vi "Prep_Config_Files_Tomography_v1.vi"() -> ()   [LabVIEW 2021]
uses:
  Pulses_char.ctl
  Drivers/Arduino_Pulse_Generator/Configurate/Channel_Pulse_Stream.ctl
  Drivers/Arduino_Pulse_Generator/Configurate/Register_1.ctl
  Drivers/Arduino_Pulse_Generator/Configurate/Register_2.ctl
  b441c710-b50f-4b81-872d-f4532ec974e2.vi
  <vilib>/Comparison/Less/Less Functor/Less Functor.lvclass
panel:
  in  "Additional mag field pumping pulse 4":T1={"Times"=[140010.0, 140020.0], "channel"=12} {"channel" min=2 max=13 step=1}
  in  "Additional mag field pumping pulse 3":T1={"Times"=[140010.0, 140020.0], "channel"=12} {"channel" min=2 max=13 step=1}
  in  "Additional mag field pumping pulse 2":T1={"Times"=[140010.0, 140020.0], "channel"=12} {"channel" min=2 max=13 step=1}
  in  "Additional mag field pumping pulse":T1={"Times"=[140010.0, 140020.0], "channel"=12} {"channel" min=2 max=13 step=1}
  out "Array - Numeric":dbl[][][][](array[numeric])
  out "Keithley TRIG":T1={"Times"=[], "channel"=2} {"channel" min=2 max=13 step=1}
  out "post_control_zy":T1={"Times"=[], "channel"=2} {"channel" min=2 max=13 step=1}
  out "post_control_non":T1={"Times"=[], "channel"=2} {"channel" min=2 max=13 step=1}
  out "post_control_y":T1={"Times"=[], "channel"=2} {"channel" min=2 max=13 step=1}
  out "post_control_z":T1={"Times"=[], "channel"=2} {"channel" min=2 max=13 step=1}
  out "control_3":T1={"Times"=[], "channel"=2} {"channel" min=2 max=13 step=1}
  out "control_2":T1={"Times"=[], "channel"=2} {"channel" min=2 max=13 step=1}
  out "control_1":T1={"Times"=[], "channel"=2} {"channel" min=2 max=13 step=1}
  out "post_cont_pulse_length":dbl
  out "control_pulse_length":dbl
  out "probe_start":dbl
  out "pump_end":dbl
  in  "Probing optical beam \nchannel":u8=2 min=2 max=13 step=1
  in  "Accqusition TRIG \nchannel":u8=6 min=2 max=13 step=1
  in  "Pumping magnetic field":T1={"Times"=[39995.0, 140005.0], "channel"=8} {"channel" min=2 max=13 step=1}
  in  "Z coil\nchannel":u8=10 min=2 max=13 step=1
  in  "Y coil\nchannel":u8=9 min=2 max=13 step=1
  in  "X coil \nchannel":u8=8 min=2 max=13 step=1
  in  "Keithley preTRIG":T1={"Times"=[2000.0, 3000.0], "channel"=5} {"channel" min=2 max=13 step=1}
  out "Accquisition TRIG":T1={"Times"=[], "channel"=2} {"channel" min=2 max=13 step=1}
  in  "Keithley ARM":T1={"Times"=[0.0, 1000.0], "channel"=4} {"channel" min=2 max=13 step=1}
  out "Probing optical beam":T1={"Times"=[], "channel"=2} {"channel" min=2 max=13 step=1}
  in  "Repumping optical beam":T1={"Times"=[40000.0, 140000.0], "channel"=3} {"channel" min=2 max=13 step=1}
  in  "Pumping optical beam":T1={"Times"=[40000.0, 140000.0], "channel"=7} {"channel" min=2 max=13 step=1}
  out "Pulses_char [ms]":T2
  in  "Z pi pulse [us]":dbl=68.0
  in  "Y pi pulse [us]":dbl=88.0
  in  "X pi pulse [us]":dbl=88.0
  # "Note that units of time are not specified there.\nRemember that minimal pulse length is about 3,8 us."
  # "channel"
  # "Control pulses"
  # "2"
  # "3"
  # "Post_control pulses"
  # "4"
  # "5"
  # "6"
  # "7"
  # "8"
  # "9"
  # "10"
  # "11"
  # "12"
  # "13"
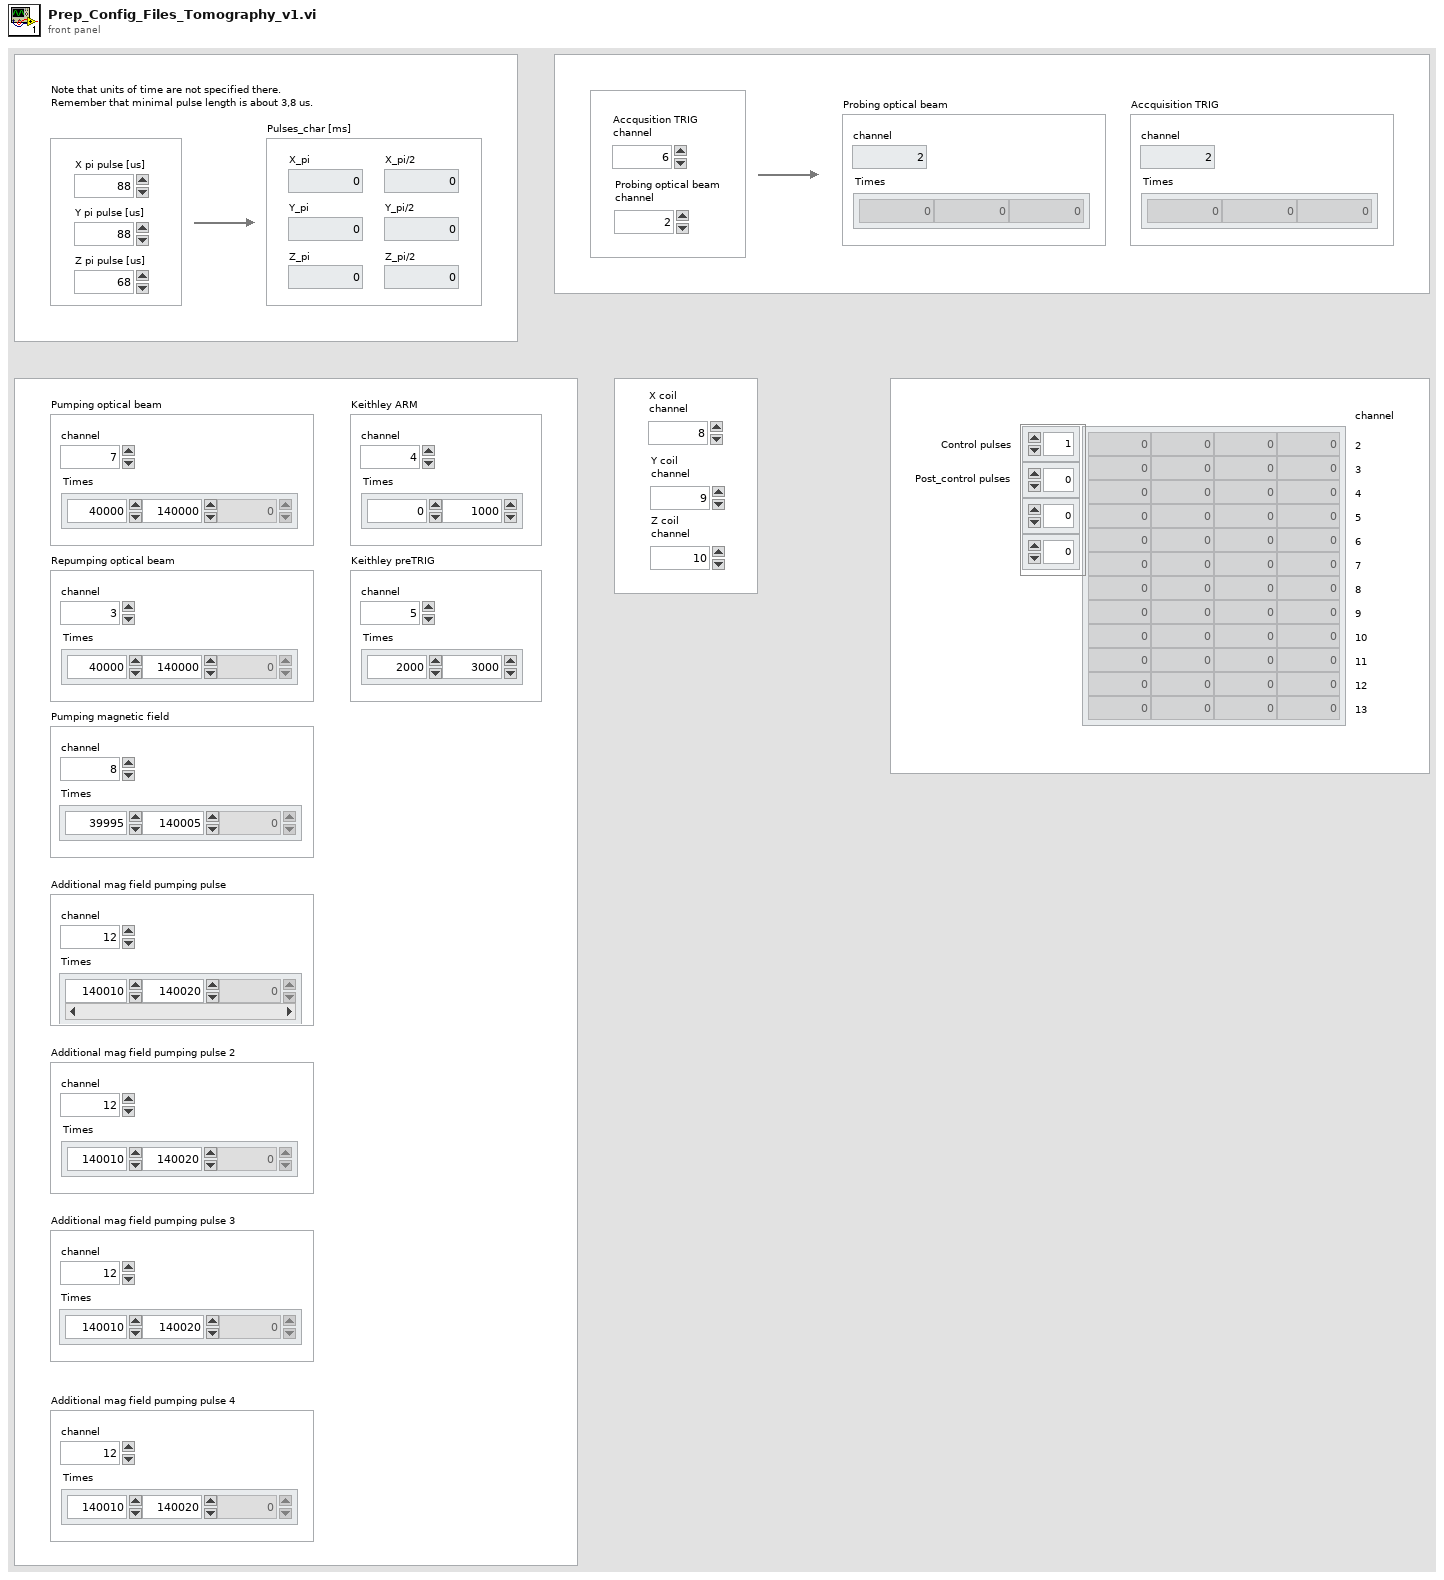
[diagram p1: front panel]
types:
  T1 = typedef "Channel_Pulse_Stream.ctl" = cluster{"Times":dbl[], "channel":u8}
  T2 = typedef "Pulses_char.ctl" = cluster{"X_pi":dbl, "Y_pi":dbl, "Z_pi":dbl, "X_pi/2":dbl, "Y_pi/2":dbl, "Z_pi/2":dbl}
  T3 = typedef "Register_2.ctl" = bool[]
  T4 = typedef "Register_1.ctl" = bool[]
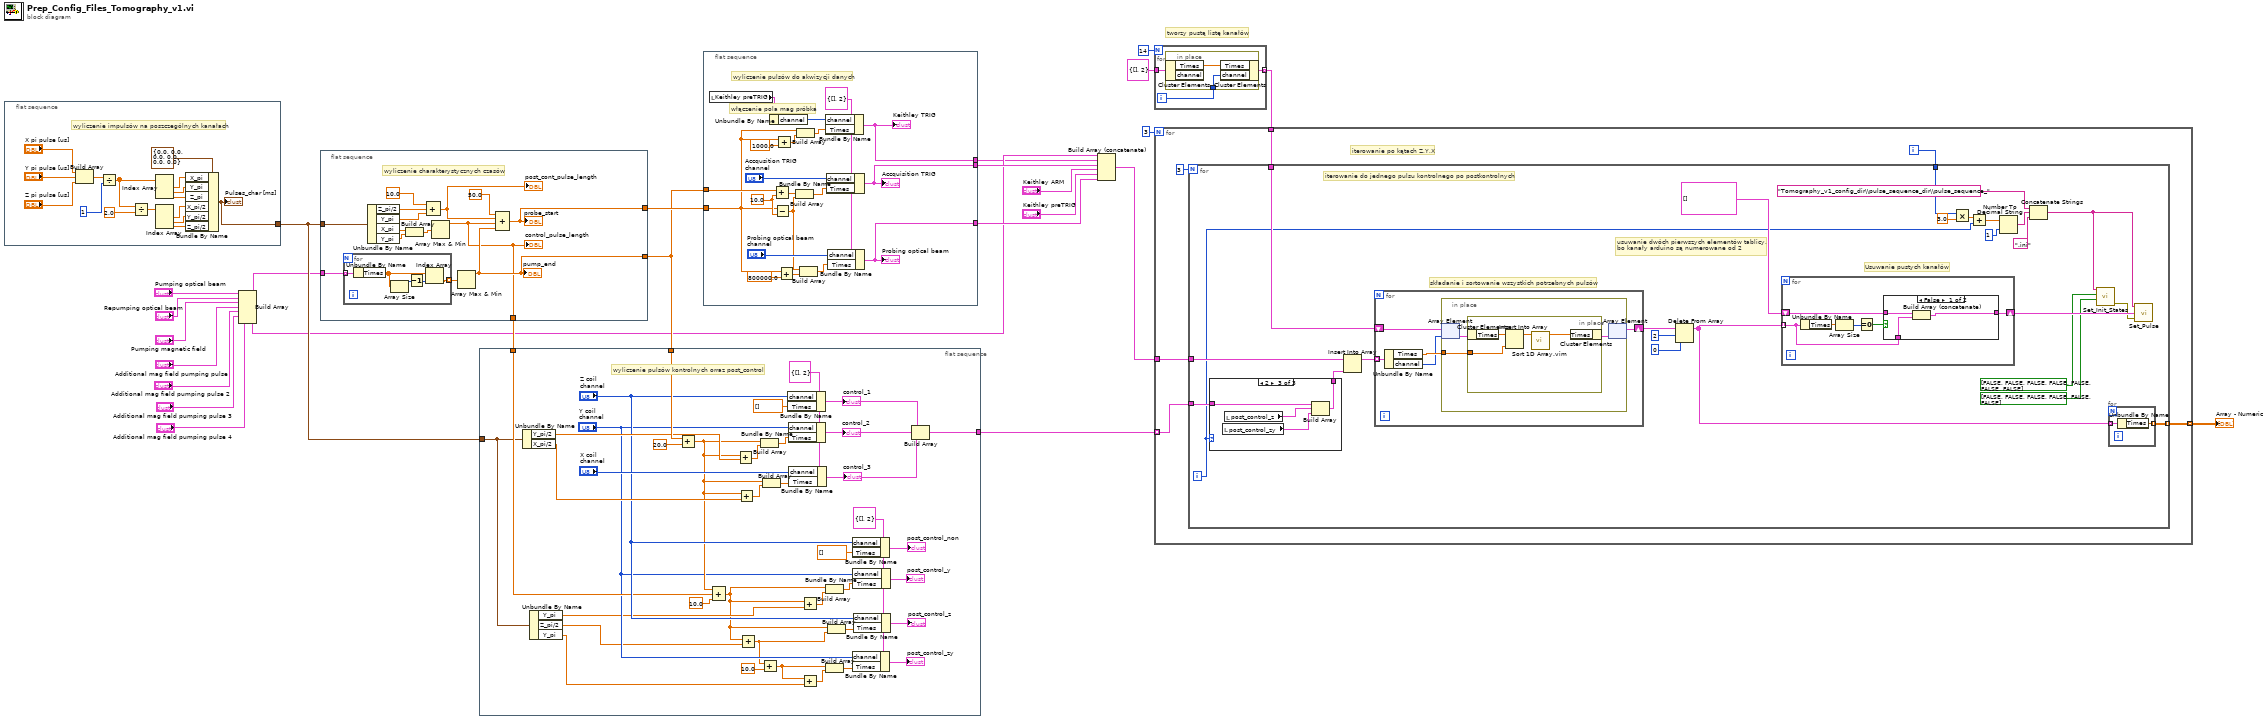
[diagram p0: block diagram]
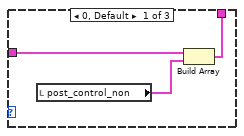
[diagram p3: hidden frame]
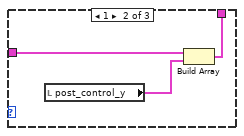
[diagram p4: hidden frame]
diagram:
  # "tworzy pustą listę kanałów"
  n1 = flat-sequence {
    tunnel: [w25] -> w18
    frame #0 {
      # "wyliczenie impulsów na poszczególnych kanałach"
      n2 = Build Array("X pi pulse [us]", "Y pi pulse [us]", "Z pi pulse [us]") -> (w40:dbl[])
      n3 = Divide(x=w40, y=1 ("Z pi pulse [us]")) -> (x/y=w32:dbl[])
      n4 = Divide(x=w32, y=2.0) -> (x/y=w33:dbl[])
      n5 = Index Array(array=w32) -> (element #1=w30:dbl, element #2=w31:dbl, element #3=w29:dbl)  [unwired: 3 in]
      n6 = Index Array(array=w33) -> (element #1=w28:dbl, element #2=w27:dbl, element #3=w26:dbl)  [unwired: 3 in]
      n7 = Bundle By Name(cluster=T2 {"X_pi"=0.0, "Y_pi"=0.0, "Z_pi"=0.0, "X_pi/2"=0.0, "Y_pi/2"=0.0, "Z_pi/2"=0.0} ("Pulses_char [ms]"), "X_pi"=w30, "Y_pi"=w31, "Z_pi"=w29, "X_pi/2"=w28, "Y_pi/2"=w27, "Z_pi/2"=w26) -> (w25:T2)
      "Pulses_char [ms]" <- w25
    }
  }
  n8 = Build Array("Pumping optical beam", "Repumping optical beam", "Pumping magnetic field", "Additional mag field pumping pulse", "Additional mag field pumping pulse 2", "Additional mag field pumping pulse 3", "Additional mag field pumping pulse 4") -> (w7:T1[])
  n9 = flat-sequence {
    tunnel: w7 -> [w54]
    tunnel: w18 -> [w49]
    tunnel: [w43] -> w20
    tunnel: [w42] -> w21
    tunnel: [w41] -> w19
    frame #0 {
      # "wyliczenie charakterystycznych czasów"
      n10 = for {
        tunnel: w54 -> [w59] mode=indexing
        tunnel: [w58] -> w53 mode=indexing
        n11 = Unbundle By Name(w59) -> ("Times"=w57:dbl[])
        n12 = Array Size(array=w57) -> (size(s)=w55:i32)
        n13 = Decrement(x=w55) -> (x-1=w56:i32)
        n14 = Index Array(array=w57, index=w56) -> (element=w58:dbl)
      }
      n15 = Unbundle By Name(w49) -> ("Z_pi/2"=w46:dbl, "Y_pi"=w47:dbl, "X_pi"=w52:dbl, "Y_pi"=w51:dbl)
      n16 = Build Array(w52, w51) -> (w50:dbl[])
      n17 = Compound Arithmetic op=ADD(10.0 ("value"), w46, w47) -> (w44:dbl)
      "post_cont_pulse_length" <- w44
      n18 = Array Max & Min(array=w50) -> (max value=w41:dbl)  [unwired: 3 out]
      "control_pulse_length" <- w41
      n19 = Array Max & Min(array=w53) -> (max value=w43:dbl)  [unwired: 3 out]
      "pump_end" <- w43
      n20 = Compound Arithmetic op=ADD(50.0 ("value"), w44, w41, w43) -> (w42:dbl)
      "probe_start" <- w42
    }
  }
  n21 = flat-sequence {
    tunnel: w20 -> [w96]
    tunnel: w19 -> [w78]
    tunnel: w18 -> [w72]
    tunnel: [w60] -> w12
    frame #0 {
      w64 = T1 {"Times"=[], "channel"=2} ("Accquisition TRIG")
      w92 = T1 {"Times"=[], "channel"=2} ("Accquisition TRIG")
      # "wyliczenie pulsów kontrolnych orraz post_control"
      n22 = Unbundle By Name(w72) -> ("Y_pi/2"=w94:dbl, "X_pi/2"=w88:dbl)
      n23 = Unbundle By Name(w72) -> ("Y_pi"=w71:dbl, "Z_pi/2"=w69:dbl, "Y_pi"=w65:dbl)
      n24 = Add(x=w96, y=20.0) -> (x+y=w79:dbl)
      n25 = Compound Arithmetic op=ADD(w79, w78, 10.0 ("value")) -> (w70:dbl)
      n26 = Add(x=w79, y=w94) -> (x+y=w93:dbl)
      n27 = Add(x=w79, y=w88) -> (x+y=w89:dbl)
      n28 = Add(x=w70, y=w69) -> (x+y=w68:dbl)
      n29 = Build Array(w79, w93) -> (w97:dbl[])
      n30 = Add(x=w68, y=10.0) -> (x+y=w66:dbl)
      n31 = Build Array(w79, w89) -> (w90:dbl[])
      n32 = Bundle By Name(cluster=w92, "channel"="Z coil\nchannel", "Times"=dbl[] []) -> (w63:T1)
      "control_1" <- w63
      n33 = Bundle By Name(cluster=w92, "channel"="Y coil\nchannel", "Times"=w97) -> (w62:T1)
      "control_2" <- w62
      n34 = Bundle By Name(cluster=w92, "channel"="X coil \nchannel", "Times"=w90) -> (w61:T1)
      "control_3" <- w61
      n35 = Add(x=w70, y=w71) -> (x+y=w85:dbl)
      n36 = Add(x=w66, y=w65) -> (x+y=w74:dbl)
      n37 = Build Array(w70, w85) -> (w84:dbl[])
      n38 = Build Array(w66, w74) -> (w75:dbl[])
      n39 = Build Array(w70, w68) -> (w87:dbl[])
      n40 = Bundle By Name(cluster=w64, "channel"="Z coil\nchannel", "Times"=dbl[] []) -> (→"post_control_non":T1)
      n41 = Bundle By Name(cluster=w64, "channel"="Y coil\nchannel", "Times"=w75) -> (→"post_control_zy":T1)
      n42 = Bundle By Name(cluster=w64, "channel"="Y coil\nchannel", "Times"=w84) -> (→"post_control_y":T1)
      n43 = Bundle By Name(cluster=w64, "channel"="Z coil\nchannel", "Times"=w87) -> (→"post_control_z":T1)
      n44 = Build Array(w63, w62, w61) -> (w60:T1[])
    }
  }
  n45 = flat-sequence {
    tunnel: w20 -> [w117]
    tunnel: w21 -> [w100]
    tunnel: [w108] -> w17
    tunnel: [w107] -> w14
    tunnel: [w102] -> w6
    frame #0 {
      w116 = 10.0 ("y")
      w106 = T1 {"Times"=[], "channel"=2} ("Accquisition TRIG")
      # "włączenie pola mag próbka"
      # "wyliczenie pulsów do akwizycji danych"
      n46 = local read "Keithley preTRIG"() -> (w105:T1)
      n47 = Unbundle By Name(w105) -> ("channel"=w104:u8)
      n48 = Add(x=w117, y=w116) -> (x+y=w115:dbl)
      n49 = Subtract(x=w100, y=w116) -> (x-y=w112:dbl)
      n50 = Add(x=w100, y=1000.0) -> (x+y=w101:dbl)
      n51 = Add(x=w100, y=800000.0) -> (x+y=w111:dbl)
      n52 = Build Array(w115, w112) -> (w114:dbl[])
      n53 = Build Array(w100, w101) -> (w103:dbl[])
      n54 = Build Array(w112, w111) -> (w109:dbl[])
      n55 = Bundle By Name(cluster=w106, "channel"=w104, "Times"=w103) -> (w102:T1)
      "Keithley TRIG" <- w102
      n56 = Bundle By Name(cluster=w106, "channel"="Accqusition TRIG \nchannel", "Times"=w114) -> (w108:T1)
      "Accquisition TRIG" <- w108
      n57 = Bundle By Name(cluster=w106, "channel"="Probing optical beam \nchannel", "Times"=w109) -> (w107:T1)
      "Probing optical beam" <- w107
    }
  }
  n58 = Build Array (concatenate)(w7, w6, w17, "Keithley ARM", "Keithley preTRIG", w14) -> (w13:T1[])
  n59 = for {
    N: 14 -> [_]
    tunnel: T1 {"Times"=[], "channel"=2} ("Channel pulse stream") -> [w121]
    tunnel: [w120] -> w8 mode=indexing
    i -> [w119]
    n60 = in-place {
      in-place-border: w119 -> [w123]
      n61 = in-place-cluster #1(w121) -> ("Times"=w122:dbl[])  [unwired: 1 out]
      n62 = in-place-cluster #1("Times"=w122, "channel"=w123) -> (w120:T1)
    }
  }
  n63 = for {
    N: 3 -> [_]
    tunnel: w13 -> [w128]
    tunnel: w12 -> [w129] mode=indexing
    tunnel: w8 -> [w126]
    tunnel: [w124] -> w5 mode=indexing
    i -> [w125]
    # "iterowanie po kątach Z,Y,X"
    n64 = for {
      N: 3 -> [_]
      tunnel: w129 -> [w154]
      tunnel: w128 -> [w153]
      tunnel: w126 -> [w150]
      tunnel: w125 -> [w139]
      tunnel: [w130] -> w124 mode=indexing
      i -> [w140]
      # "Usuwanie pustych kanałów"
      # "usuwanie dwóch pierwszych elementów tablicy, \nbo kanały arduino są numerowane od 2"
      # "składanie i sortowanie wszystkich potrzebnych pulsów"
      # "iterowanie do jednego pulsu kontrolnego po postkontrolnych"
      n65 = case shown="2" w140 {
        tunnel: w154 -> [w181 w184 w188]
        tunnel: [w179 w182 w185] -> w152
        frame 0, Default {
          n66 = local read "post_control_non"() -> (w180:T1)
          n67 = Build Array(w181, w180) -> (w179:T1[])
        }
        frame 1 {
          n68 = local read "post_control_y"() -> (w183:T1)
          n69 = Build Array(w184, w183) -> (w182:T1[])
        }
        frame 2 {
          n70 = local read "post_control_zy"() -> (w186:T1)
          n71 = local read "post_control_z"() -> (w187:T1)
          n72 = Build Array(w188, w187, w186) -> (w185:T1[])
        }
      }
      n73 = Insert Into Array(array=w153, new element=w152) -> (w151:T1[])  [unwired: 1 in]
      n74 = for {
        tunnel: w151 -> [w171] mode=indexing
        shift-right: [w167] -> w147
        shift-left: w150 -> [w169]
        n75 = Unbundle By Name(w171) -> ("Times"=w170:dbl[], "channel"=w168:u8)
        n76 = in-place {
          in-place-border: w170 -> [w174]
          n77 = in-place-array #2(w169, w168) -> (w172:T1)
          n78 = in-place {
            in-place-border: w174 -> [w177]
            n79 = in-place-cluster #3(w172) -> ("Times"=w178:dbl[])
            n80 = Insert Into Array(array=w178, new element=w177) -> (w176:dbl[])  [unwired: 1 in]
            n81 = call "Sort 1D Array.vim"("unsorted array"=w176) -> ("sorted array"=w175:dbl[])  [unwired: 10 in]
            n82 = in-place-cluster #3("Times"=w175) -> (w173:T1)
          }
          n83 = in-place-array #2(w173) -> (w167:T1[])  [unwired: 1 out]
        }
      }
      n84 = Delete From Array(array=w147, length=2, index=0) -> (array with subset deleted=w145:T1[])  [unwired: 1 out]
      n85 = for {
        shift-right: [w157] -> w135
        shift-left: T1[] [] -> [w156]
        tunnel: w145 -> [w155] mode=indexing
        n86 = Unbundle By Name(w155) -> ("Times"=w160:dbl[])
        n87 = Array Size(array=w160) -> (size(s)=w159:i32)
        n88 = Equal To 0?(x=w159) -> (x = 0?=w158:bool)
        n89 = case shown="False" w158 {
          tunnel: w156 -> [w163 w164]
          tunnel: [w161 w164] -> w157
          tunnel: w155 -> [w162 _]
          frame False {
            n90 = Build Array (concatenate)(w163, w162) -> (w161:T1[])
          }
          frame True {
          }
        }
      }
      n91 = Multiply(x=w139, y=3.0) -> (x*y=w141:dbl)
      n92 = Add(x=w141, y=w140) -> (x+y=w138:dbl)
      n93 = Number To Decimal String(number=w138, width (-)=i16 1) -> (decimal integer string=w143:string)
      n94 = Concatenate Strings("Tomography_v1_config_dir\\pulse_sequence_dir\\pulse_sequence_" ("Filename (.ini)"), w143, ".ini" ("string")) -> (w133:string)
      n95 = call "Set_Init_States.vi"("register 2 (8-13)"=T3 [FALSE, FALSE, FALSE, FALSE, FALSE, FALSE], "register 1 (2-7)"=T4 [FALSE, FALSE, FALSE, FALSE, FALSE, FALSE, FALSE], "Filename (ini)"=w133) -> ("error out"=w134:errorcluster)  [unwired: 4 in]
      n96 = for {
        tunnel: w145 -> [w166] mode=indexing
        tunnel: [w165] -> w130 mode=indexing
        n97 = Unbundle By Name(w166) -> ("Times"=w165:dbl[])
      }
      n98 = call "Set_Pulse.vi"("error in"=w134, "Pulse sequence"=w135, "Filename (.ini)"=w133) -> ()  [unwired: 1 in, 1 out]
    }
  }
  "Array - Numeric" <- w5
